vi "DownsampleStage2_5160_singlechannel.vi"(7 "reset":bool, 8 "valid in":bool, 10 "I in":fxp<+/-,16,14>, 11 "Q in":fxp<+/-,16,14>) -> (0 "valid out":bool, 3 "IQ out":u32)   [LabVIEW 2013]
uses:
  <vilib>/rvi/FXPMathLib/FxpInterpret/XNode/nifxpmath_Interpret.xnode
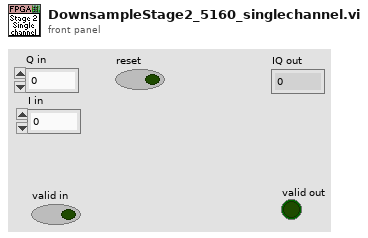
[diagram p1: front panel]
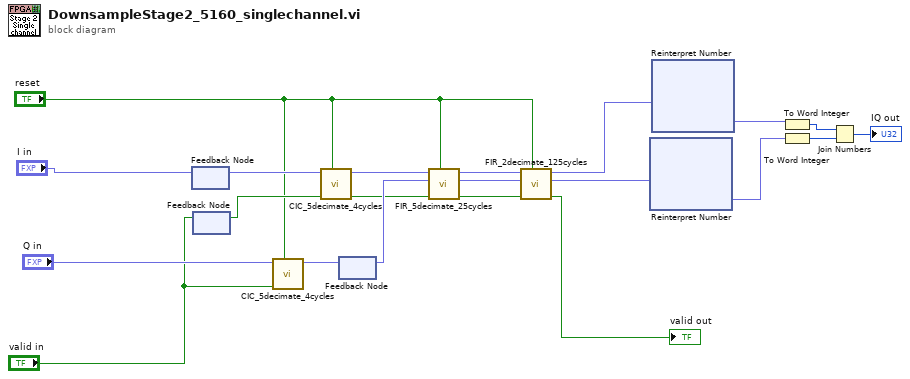
[diagram p0: block diagram]
diagram:
  n1 = feedback #1() -> (w21:fxp<+/-,16,14>)  [unwired: 1 in]
  n2 = feedback-in #1("I in") -> ()
  n3 = feedback #2() -> (w20:bool)  [unwired: 1 in]
  n4 = feedback-in #2("valid in") -> ()
  n5 = call "CIC_5decimate_4cycles.vi"("reset"="reset", "valid in"="valid in", "Data in"="Q in") -> ("Data out"=w18:fxp<+/-,16,14>)  [unwired: 6 in, 2 out]
  n6 = call "CIC_5decimate_4cycles.vi"("reset"="reset", "valid in"=w20, "Data in"=w21) -> ("valid out"=w15:bool, "Data out"=w17:fxp<+/-,16,14>)  [unwired: 6 in, 1 out]
  n7 = feedback #3() -> (w16:fxp<+/-,16,14>)  [unwired: 1 in]
  n8 = feedback-in #3(w18) -> ()
  n9 = call "FIR_5decimate_25cycles.vi"("reset"="reset", "valid in"=w15, "Q in"=w16, "I in"=w17) -> ("valid out"=w1:bool, "Q out"=w2:fxp<+/-,16,14>, "I out"=w3:fxp<+/-,16,14>)  [unwired: 4 in, 1 out]
  n10 = call "FIR_2decimate_125cycles.vi"("reset"="reset", "valid in"=w1, "Q in"=w2, "I in"=w3) -> ("valid out"=→"valid out":bool, "Q out"=w7:fxp<+/-,16,14>, "I out"=w6:fxp<+/-,16,14>)  [unwired: 4 in, 1 out]
  n11 = xnode "Reinterpret Number"("x"=w7) -> ("y"=w4:fxp<+/-,16,16>)
  n12 = xnode "Reinterpret Number"("x"=w6) -> ("y"=w5:fxp<+/-,16,16>)
  n13 = To Word Integer(number=w5) -> (16bit integer=w9:i16)
  n14 = To Word Integer(number=w4) -> (16bit integer=w10:i16)
  n15 = Join Numbers(hi=w9, lo=w10) -> ((hi.lo)=→"IQ out":u32)
